vi "Throttle.vi"(0 "Up":bool, 5 "Down":bool, 7 "X (IN)":dbl, 9 "Y (IN)":dbl, 11 "Rotation (IN)":dbl) -> (6 "Throttle":dbl, 8 "X (OUT)":dbl, 10 "Y (OUT)":dbl, 15 "Rotation (OUT)":dbl)   [LabVIEW 2014]
uses:
  Robot Global Data.vi
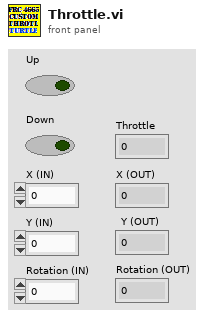
[diagram p1: front panel]
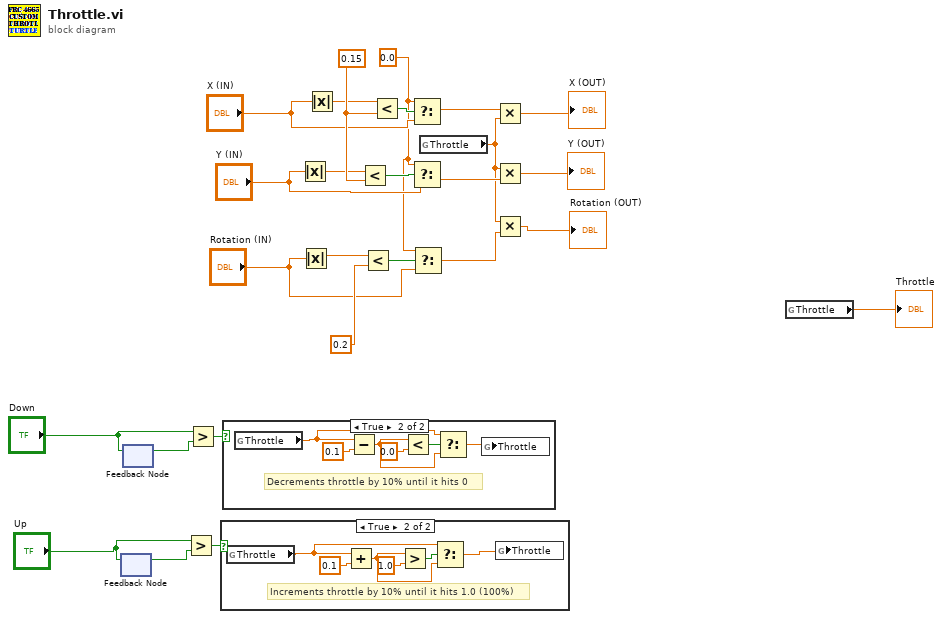
[diagram p0: block diagram]
diagram:
  w4 = 0.0
  w25 = 0.15
  n1 = feedback #1() -> (w15:bool)  [unwired: 1 in]
  n2 = feedback-in #1("Up") -> ()
  n3 = feedback #2() -> (w16:bool)  [unwired: 1 in]
  n4 = feedback-in #2("Down") -> ()
  n5 = Greater?(x="Up", y=w15) -> (0:w14:bool)
  n6 = Greater?(x="Down", y=w16) -> (0:w17:bool)
  n7 = case shown="True" w14 {
    frame False {
    }
    frame True {
      # "Increments throttle by 10% until it hits 1.0 (100%)"
      n8 = global read "Robot Global Data.vi" "Throttle"() -> (w28:dbl)
      n9 = Add(x=w28, y=0.1) -> (x+y=w29:dbl)
      n10 = Greater?(x=w29, y=1.0) -> (0:w30:bool)
      n11 = Select(t=w28, s=w30, f=w29) -> (s? t:f=w27:dbl)
      n12 = global write "Robot Global Data.vi" "Throttle"(w27) -> ()
    }
  }
  n13 = case shown="True" w17 {
    frame False {
    }
    frame True {
      # "Decrements throttle by 10% until it hits 0"
      n14 = global read "Robot Global Data.vi" "Throttle"() -> (w34:dbl)
      n15 = Subtract(x=w34, y=0.1) -> (x-y=w36:dbl)
      n16 = Less?(x=w36, y=0.0) -> (x < y?=w37:bool)
      n17 = Select(t=w34, s=w37, f=w36) -> (s? t:f=w33:dbl)
      n18 = global write "Robot Global Data.vi" "Throttle"(w33) -> ()
    }
  }
  n19 = Absolute Value(x="Y (IN)") -> (abs(x)=w24:dbl)
  n20 = Absolute Value(x="Rotation (IN)") -> (abs(x)=w5:dbl)
  n21 = Absolute Value(x="X (IN)") -> (abs(x)=w23:dbl)
  n22 = Less?(x=w24, y=w25) -> (x < y?=w22:bool)
  n23 = Less?(x=w5, y=0.2) -> (x < y?=w19:bool)
  n24 = Less?(x=w23, y=w25) -> (x < y?=w26:bool)
  n25 = Select(t=w4, s=w26, f="X (IN)") -> (s? t:f=w20:dbl)
  n26 = Select(t=w4, s=w22, f="Y (IN)") -> (s? t:f=w21:dbl)
  n27 = Select(t=w4, s=w19, f="Rotation (IN)") -> (s? t:f=w3:dbl)
  n28 = global read "Robot Global Data.vi" "Throttle"() -> (w2:dbl)
  n29 = Multiply(x=w20, y=w2) -> (x*y=→"X (OUT)":dbl)
  n30 = Multiply(x=w2, y=w21) -> (x*y=→"Y (OUT)":dbl)
  n31 = Multiply(x=w2, y=w3) -> (x*y=→"Rotation (OUT)":dbl)
  n32 = global read "Robot Global Data.vi" "Throttle"() -> (→"Throttle":dbl)
